vi "CAN Jaguar Get Status.vi"(8 "error in (no error)":errorcluster, 10 "Status Select":T1[](array[typedef])=[enum."Voltage"], 11 "CAN Jaguar Ref":T3={"Device Number"=0, "Control Mode"=enum."Percent VBus", "Inverted"=FALSE, "Semaphore"=refnum, "Max Vout"=12.0, "DevStatus"={"status"=FALSE, "code"=0, "source"=""}}) -> (0 "error out":errorcluster, 2 "Status":T2, 3 "CAN Jaguar Ref Out":T3={"Device Number"=0, "Control Mode"=enum."Percent VBus", "Inverted"=FALSE, "Semaphore"=refnum, "Max Vout"=12.0, "DevStatus"={"status"=FALSE, "code"=0, "source"=""}})   [LabVIEW 2009, in "CAN.lvlib"]
uses:
  CAN.lvlib
  SubVIs/CAN Jaguar Ref.ctl
  SubVIs/CAN Jaguar Control Mode.ctl
  SubVIs/CAN Jaguar Status.ctl
  SubVIs/CAN Jaguar Status Select.ctl
  SubVIs/CAN Motor Message IDs.ctl
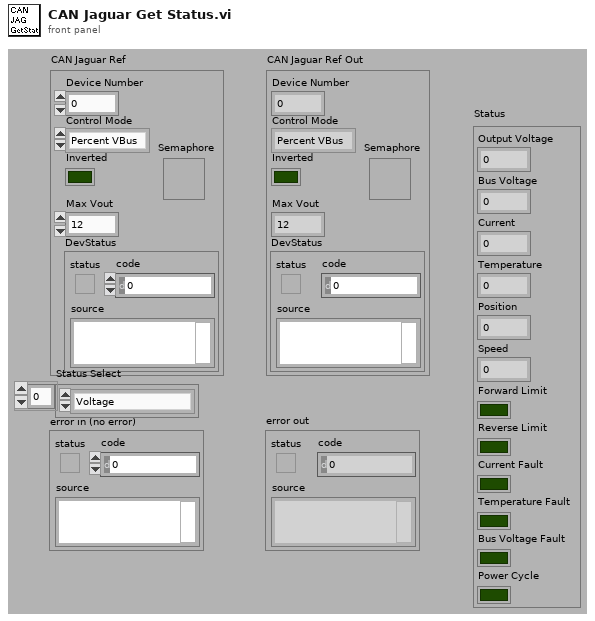
[diagram p1: front panel]
types:
  T1 = typedef "CAN.lvlib/CAN Jaguar Status Select.ctl" = enum16{"Voltage", "Current", "Temperature", "Position", "Speed", "Limit Switches", "Faults", "Power Cycle"}
  T2 = typedef "CAN.lvlib/CAN Jaguar Status.ctl" = cluster{"Output Voltage":dbl, "Bus Voltage":dbl, "Current":dbl, "Temperature":dbl, "Position":dbl, "Speed":dbl, "Forward Limit":bool, "Reverse Limit":bool, "Current Fault":bool, "Temperature Fault":bool, "Bus Voltage Fault":bool, "Power Cycle":bool}
  T3 = typedef "CAN.lvlib/CAN Jaguar Ref.ctl" = cluster{"Device Number":u8, "Control Mode":T4, "Inverted":bool, "Semaphore":T5, "Max Vout":dbl, "DevStatus":errorcluster}
  T4 = typedef "CAN.lvlib/CAN Jaguar Control Mode.ctl" = enum16{"Percent VBus", "Speed", "Position", "Current"}
  T5 = typedef "Semaphore RefNum" = refnum<k1>
  T6 = enum16{"big-endian, network order", "native, host order", "little-endian"}
  T7 = typedef "CAN Jaguar Status.ctl" = cluster{"Output Voltage":dbl, "Bus Voltage":dbl, "Current":dbl, "Temperature":dbl, "Position":dbl, "Speed":dbl, "Forward Limit":bool, "Reverse Limit":bool, "Current Fault":bool, "Temperature Fault":bool, "Bus Voltage Fault":bool, "Power Cycle":bool}
  T8 = typedef "CAN.lvlib/CAN Motor Message IDs.ctl" = u32
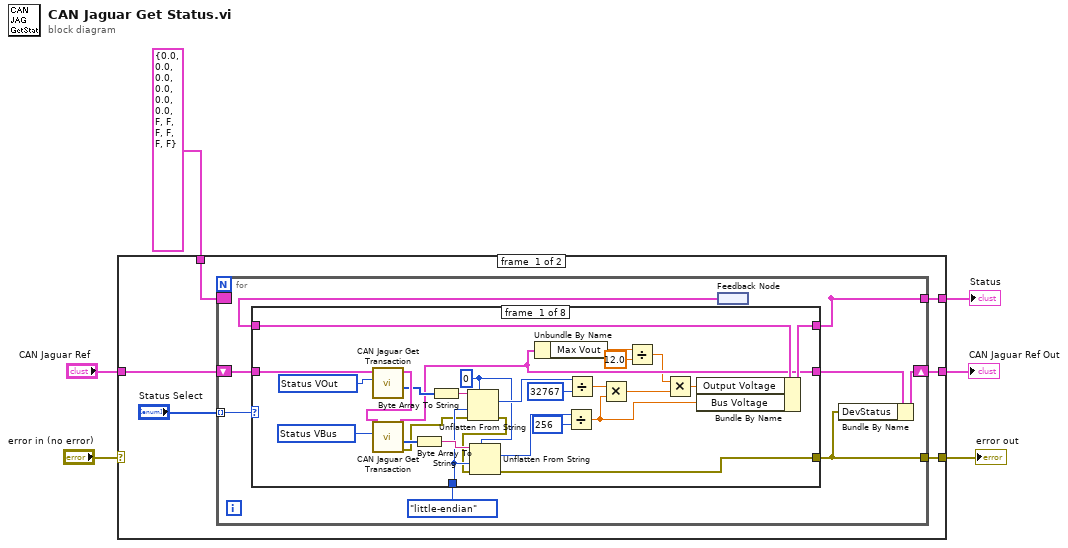
[diagram p0: block diagram]
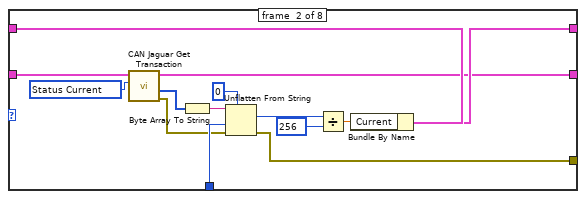
[diagram p2: hidden frame]
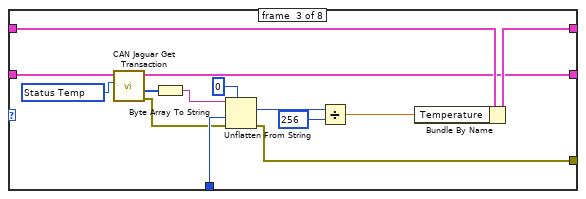
[diagram p3: hidden frame]
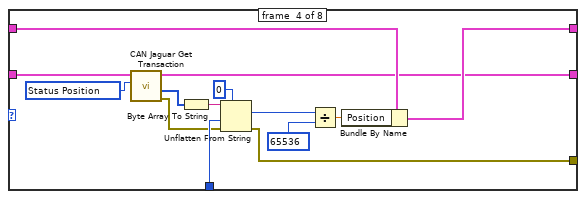
[diagram p4: hidden frame]
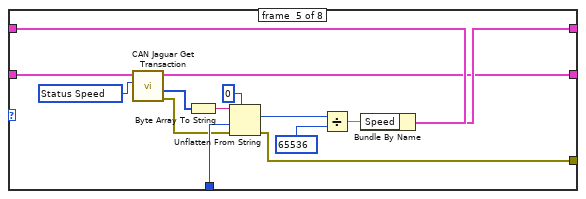
[diagram p5: hidden frame]
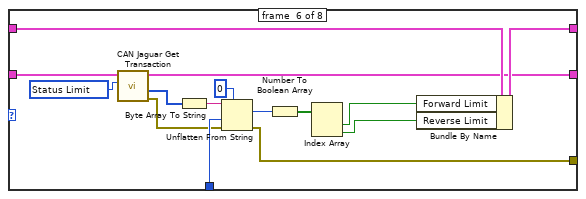
[diagram p6: hidden frame]
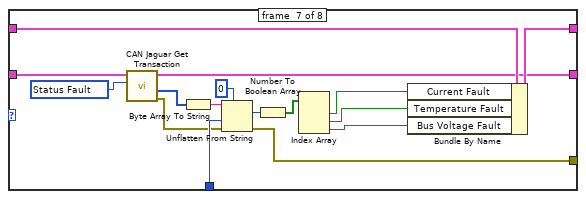
[diagram p7: hidden frame]
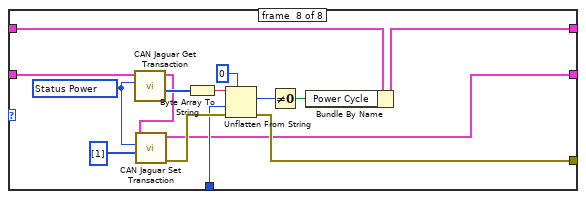
[diagram p8: hidden frame]
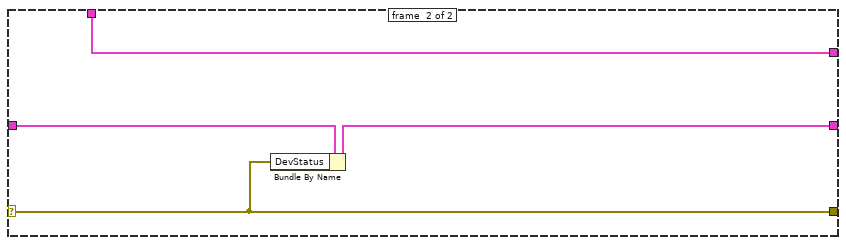
[diagram p9: hidden frame]
diagram:
  n1 = case shown="No Error" "error in (no error)" {
    selector: "error in (no error)" -> [_ w151]
    tunnel: [w7 w152] -> w6
    tunnel: "CAN Jaguar Ref" -> [w8 w153]
    tunnel: [w12 w151] -> w4
    tunnel: T2 {"Output Voltage"=0.0, "Bus Voltage"=0.0, "Current"=0.0, "Temperature"=0.0, "Position"=0.0, "Speed"=0.0, "Forward Limit"=FALSE, "Reverse Limit"=FALSE, "Current Fault"=FALSE, "Temperature Fault"=FALSE, "Bus Voltage Fault"=FALSE, "Power Cycle"=FALSE} ("Status") -> [w10 w150]
    tunnel: [w9 w150] -> w1
    frame #0 {
      n2 = for {
        tunnel: [w15] -> w12
        tunnel: "Status Select" -> [w20] mode=indexing
        border: w10 -> [_]
        tunnel: [w17] -> w9
        shift-right: [w13] -> w7
        shift-left: w8 -> [w16]
        n3 = feedback #1() -> (w19:T7)
        n4 = case shown="\"Voltage\"" w20 {
          tunnel: T6."little-endian" ("byte order (0:big-endian, network order)") -> [w29 w61 w75 w89 w103 w118 w134 w137]
          tunnel: [w47 w59 w73 w87 w101 w116 w132 w138] -> w15
          tunnel: w19 -> [w45 w58 w70 w86 w100 w115 w131 w149]
          tunnel: [w44 w57 w69 w85 w99 w114 w130 w148] -> w17
          tunnel: w16 -> [w34 w50 w67 w77 w91 w106 w121 w139]
          tunnel: [w25 w48 w62 w76 w90 w104 w119 w135] -> w14
          frame #0 {
            w27 = i16 0 ("Voltage")
            w35 = T8 33690624 items=["Volt Enable"=33685504, "Volt Disable"=33685568, "Volt Set"=33685632, "Volt Set Ramp"=33685696, "Speed Enable"=33686528, "Speed Disable"=33686592, "Speed Set"=33686656, "Speed P"=33686720, "Speed I"=33686784, "Speed D"=33686848, "Speed Ref"=33686912, "Position Enable"=33688576, "Position Disable"=33688640, "Position Set"=33688704, "Position P"=33688768, "Position I"=33688832, "Position D"=33688896, "Position Ref"=33688960, "Current Enable"=33689600, "Current Disable"=33689664, "Current Set"=33689728, "Current P"=33689792, "Current I"=33689856, "Current D"=33689920, "Status VOut"=33690624, "Status VBus"=33690688, "Status Current"=33690752, "Status Temp"=33690816, "Status Position"=33690880, "Status Speed"=33690944, "Status Limit"=33691008, "Status Fault"=33691072, "Status Power"=33691136, "Config Num Brushes"=33692672, "Config Encoder Lines"=33692736, "Config Pot Turns"=33692800, "Config Brake Coast"=33692864, "Config Limit Mode"=33692928, "Config Limit Fwd"=33692992, "Config Limit Rev"=33693056, "Config Max VOut"=33693120, "Config Fault Time"=33693184, "Motor Ack"=33693696] ("CAN Motor Message IDs")
            w36 = T8 33690688 items=["Volt Enable"=33685504, "Volt Disable"=33685568, "Volt Set"=33685632, "Volt Set Ramp"=33685696, "Speed Enable"=33686528, "Speed Disable"=33686592, "Speed Set"=33686656, "Speed P"=33686720, "Speed I"=33686784, "Speed D"=33686848, "Speed Ref"=33686912, "Position Enable"=33688576, "Position Disable"=33688640, "Position Set"=33688704, "Position P"=33688768, "Position I"=33688832, "Position D"=33688896, "Position Ref"=33688960, "Current Enable"=33689600, "Current Disable"=33689664, "Current Set"=33689728, "Current P"=33689792, "Current I"=33689856, "Current D"=33689920, "Status VOut"=33690624, "Status VBus"=33690688, "Status Current"=33690752, "Status Temp"=33690816, "Status Position"=33690880, "Status Speed"=33690944, "Status Limit"=33691008, "Status Fault"=33691072, "Status Power"=33691136, "Config Num Brushes"=33692672, "Config Encoder Lines"=33692736, "Config Pot Turns"=33692800, "Config Brake Coast"=33692864, "Config Limit Mode"=33692928, "Config Limit Fwd"=33692992, "Config Limit Rev"=33693056, "Config Max VOut"=33693120, "Config Fault Time"=33693184, "Motor Ack"=33693696] ("CAN Motor Message IDs")
            n5 = call "CAN Jaguar Get Transaction.vi"("Message ID"=w35, "CAN Jaguar Ref"=w34) -> ("Data"=w31:u8[], "CAN Jaguar Ref Out"=w33:T3)  [unwired: 1 in, 7 out]
            n6 = call "CAN Jaguar Get Transaction.vi"("Message ID"=w36, "CAN Jaguar Ref"=w33) -> ("error out"=w28:errorcluster, "Data"=w37:u8[], "CAN Jaguar Ref Out"=w25:T3)  [unwired: 1 in, 6 out]
            n7 = Byte Array To String(unsigned byte array=w37) -> (string=w38:string)
            n8 = Byte Array To String(unsigned byte array=w31) -> (string=w32:string)
            n9 = Unflatten From String(type=w27, binary string=w32, byte order (0:big-endian, network order)=w29, error in (no error)=w28) -> (value=w30:i16, error out=w26:errorcluster)  [unwired: 2 out]
            n10 = Unflatten From String(type=w27, binary string=w38, byte order (0:big-endian, network order)=w29, error in (no error)=w26) -> (value=w43:i16, error out=w47:errorcluster)  [unwired: 2 out]
            n11 = Unbundle By Name(w25) -> ("Max Vout"=w23:dbl)
            n12 = Divide(x=w43, y=i16 256) -> (x/y=w40:dbl)
            n13 = Divide(x=w30, y=i16 32767) -> (x/y=w39:dbl)
            n14 = Multiply(x=w39, y=w40) -> (x*y=w41:dbl)
            n15 = Divide(x=w23, y=12.0) -> (x/y=w21:dbl)
            n16 = Multiply(x=w21, y=w41) -> (x*y=w24:dbl)
            n17 = Bundle By Name(cluster=w45, "Output Voltage"=w24, "Bus Voltage"=w40) -> (w44:T7)
          }
          frame #1 {
            w49 = T8 33690752 items=["Volt Enable"=33685504, "Volt Disable"=33685568, "Volt Set"=33685632, "Volt Set Ramp"=33685696, "Speed Enable"=33686528, "Speed Disable"=33686592, "Speed Set"=33686656, "Speed P"=33686720, "Speed I"=33686784, "Speed D"=33686848, "Speed Ref"=33686912, "Position Enable"=33688576, "Position Disable"=33688640, "Position Set"=33688704, "Position P"=33688768, "Position I"=33688832, "Position D"=33688896, "Position Ref"=33688960, "Current Enable"=33689600, "Current Disable"=33689664, "Current Set"=33689728, "Current P"=33689792, "Current I"=33689856, "Current D"=33689920, "Status VOut"=33690624, "Status VBus"=33690688, "Status Current"=33690752, "Status Temp"=33690816, "Status Position"=33690880, "Status Speed"=33690944, "Status Limit"=33691008, "Status Fault"=33691072, "Status Power"=33691136, "Config Num Brushes"=33692672, "Config Encoder Lines"=33692736, "Config Pot Turns"=33692800, "Config Brake Coast"=33692864, "Config Limit Mode"=33692928, "Config Limit Fwd"=33692992, "Config Limit Rev"=33693056, "Config Max VOut"=33693120, "Config Fault Time"=33693184, "Motor Ack"=33693696] ("CAN Motor Message IDs")
            n18 = call "CAN Jaguar Get Transaction.vi"("Message ID"=w49, "CAN Jaguar Ref"=w50) -> ("error out"=w51:errorcluster, "Data"=w52:u8[], "CAN Jaguar Ref Out"=w48:T3)  [unwired: 1 in, 6 out]
            n19 = Byte Array To String(unsigned byte array=w52) -> (string=w53:string)
            n20 = Unflatten From String(type=i16 0 ("Voltage"), binary string=w53, byte order (0:big-endian, network order)=w61, error in (no error)=w51) -> (value=w56:i16, error out=w59:errorcluster)  [unwired: 2 out]
            n21 = Divide(x=w56, y=256) -> (x/y=w54:dbl)
            n22 = Bundle By Name(cluster=w58, "Current"=w54) -> (w57:T7)
          }
          frame #2 {
            w64 = T8 33690816 items=["Volt Enable"=33685504, "Volt Disable"=33685568, "Volt Set"=33685632, "Volt Set Ramp"=33685696, "Speed Enable"=33686528, "Speed Disable"=33686592, "Speed Set"=33686656, "Speed P"=33686720, "Speed I"=33686784, "Speed D"=33686848, "Speed Ref"=33686912, "Position Enable"=33688576, "Position Disable"=33688640, "Position Set"=33688704, "Position P"=33688768, "Position I"=33688832, "Position D"=33688896, "Position Ref"=33688960, "Current Enable"=33689600, "Current Disable"=33689664, "Current Set"=33689728, "Current P"=33689792, "Current I"=33689856, "Current D"=33689920, "Status VOut"=33690624, "Status VBus"=33690688, "Status Current"=33690752, "Status Temp"=33690816, "Status Position"=33690880, "Status Speed"=33690944, "Status Limit"=33691008, "Status Fault"=33691072, "Status Power"=33691136, "Config Num Brushes"=33692672, "Config Encoder Lines"=33692736, "Config Pot Turns"=33692800, "Config Brake Coast"=33692864, "Config Limit Mode"=33692928, "Config Limit Fwd"=33692992, "Config Limit Rev"=33693056, "Config Max VOut"=33693120, "Config Fault Time"=33693184, "Motor Ack"=33693696] ("CAN Motor Message IDs")
            n23 = call "CAN Jaguar Get Transaction.vi"("Message ID"=w64, "CAN Jaguar Ref"=w67) -> ("error out"=w63:errorcluster, "Data"=w66:u8[], "CAN Jaguar Ref Out"=w62:T3)  [unwired: 1 in, 6 out]
            n24 = Byte Array To String(unsigned byte array=w66) -> (string=w65:string)
            n25 = Unflatten From String(type=i16 0 ("Voltage"), binary string=w65, byte order (0:big-endian, network order)=w75, error in (no error)=w63) -> (value=w72:i16, error out=w73:errorcluster)  [unwired: 2 out]
            n26 = Divide(x=w72, y=256) -> (x/y=w68:dbl)
            n27 = Bundle By Name(cluster=w70, "Temperature"=w68) -> (w69:T7)
          }
          frame #3 {
            w80 = T8 33690880 items=["Volt Enable"=33685504, "Volt Disable"=33685568, "Volt Set"=33685632, "Volt Set Ramp"=33685696, "Speed Enable"=33686528, "Speed Disable"=33686592, "Speed Set"=33686656, "Speed P"=33686720, "Speed I"=33686784, "Speed D"=33686848, "Speed Ref"=33686912, "Position Enable"=33688576, "Position Disable"=33688640, "Position Set"=33688704, "Position P"=33688768, "Position I"=33688832, "Position D"=33688896, "Position Ref"=33688960, "Current Enable"=33689600, "Current Disable"=33689664, "Current Set"=33689728, "Current P"=33689792, "Current I"=33689856, "Current D"=33689920, "Status VOut"=33690624, "Status VBus"=33690688, "Status Current"=33690752, "Status Temp"=33690816, "Status Position"=33690880, "Status Speed"=33690944, "Status Limit"=33691008, "Status Fault"=33691072, "Status Power"=33691136, "Config Num Brushes"=33692672, "Config Encoder Lines"=33692736, "Config Pot Turns"=33692800, "Config Brake Coast"=33692864, "Config Limit Mode"=33692928, "Config Limit Fwd"=33692992, "Config Limit Rev"=33693056, "Config Max VOut"=33693120, "Config Fault Time"=33693184, "Motor Ack"=33693696] ("CAN Motor Message IDs")
            n28 = call "CAN Jaguar Get Transaction.vi"("Message ID"=w80, "CAN Jaguar Ref"=w77) -> ("error out"=w79:errorcluster, "Data"=w78:u8[], "CAN Jaguar Ref Out"=w76:T3)  [unwired: 1 in, 6 out]
            n29 = Byte Array To String(unsigned byte array=w78) -> (string=w81:string)
            n30 = Unflatten From String(type=0 ("Voltage"), binary string=w81, byte order (0:big-endian, network order)=w89, error in (no error)=w79) -> (value=w84:i32, error out=w87:errorcluster)  [unwired: 2 out]
            n31 = Divide(x=w84, y=65536 ("value")) -> (x/y=w83:dbl)
            n32 = Bundle By Name(cluster=w86, "Position"=w83) -> (w85:T7)
          }
          frame #4 {
            w92 = T8 33690944 items=["Volt Enable"=33685504, "Volt Disable"=33685568, "Volt Set"=33685632, "Volt Set Ramp"=33685696, "Speed Enable"=33686528, "Speed Disable"=33686592, "Speed Set"=33686656, "Speed P"=33686720, "Speed I"=33686784, "Speed D"=33686848, "Speed Ref"=33686912, "Position Enable"=33688576, "Position Disable"=33688640, "Position Set"=33688704, "Position P"=33688768, "Position I"=33688832, "Position D"=33688896, "Position Ref"=33688960, "Current Enable"=33689600, "Current Disable"=33689664, "Current Set"=33689728, "Current P"=33689792, "Current I"=33689856, "Current D"=33689920, "Status VOut"=33690624, "Status VBus"=33690688, "Status Current"=33690752, "Status Temp"=33690816, "Status Position"=33690880, "Status Speed"=33690944, "Status Limit"=33691008, "Status Fault"=33691072, "Status Power"=33691136, "Config Num Brushes"=33692672, "Config Encoder Lines"=33692736, "Config Pot Turns"=33692800, "Config Brake Coast"=33692864, "Config Limit Mode"=33692928, "Config Limit Fwd"=33692992, "Config Limit Rev"=33693056, "Config Max VOut"=33693120, "Config Fault Time"=33693184, "Motor Ack"=33693696] ("CAN Motor Message IDs")
            n33 = call "CAN Jaguar Get Transaction.vi"("Message ID"=w92, "CAN Jaguar Ref"=w91) -> ("error out"=w93:errorcluster, "Data"=w94:u8[], "CAN Jaguar Ref Out"=w90:T3)  [unwired: 1 in, 6 out]
            n34 = Byte Array To String(unsigned byte array=w94) -> (string=w95:string)
            n35 = Unflatten From String(type=0 ("Voltage"), binary string=w95, byte order (0:big-endian, network order)=w103, error in (no error)=w93) -> (value=w96:i32, error out=w101:errorcluster)  [unwired: 2 out]
            n36 = Divide(x=w96, y=65536 ("value")) -> (x/y=w97:dbl)
            n37 = Bundle By Name(cluster=w100, "Speed"=w97) -> (w99:T7)
          }
          frame #5 {
            w105 = T8 33691008 items=["Volt Enable"=33685504, "Volt Disable"=33685568, "Volt Set"=33685632, "Volt Set Ramp"=33685696, "Speed Enable"=33686528, "Speed Disable"=33686592, "Speed Set"=33686656, "Speed P"=33686720, "Speed I"=33686784, "Speed D"=33686848, "Speed Ref"=33686912, "Position Enable"=33688576, "Position Disable"=33688640, "Position Set"=33688704, "Position P"=33688768, "Position I"=33688832, "Position D"=33688896, "Position Ref"=33688960, "Current Enable"=33689600, "Current Disable"=33689664, "Current Set"=33689728, "Current P"=33689792, "Current I"=33689856, "Current D"=33689920, "Status VOut"=33690624, "Status VBus"=33690688, "Status Current"=33690752, "Status Temp"=33690816, "Status Position"=33690880, "Status Speed"=33690944, "Status Limit"=33691008, "Status Fault"=33691072, "Status Power"=33691136, "Config Num Brushes"=33692672, "Config Encoder Lines"=33692736, "Config Pot Turns"=33692800, "Config Brake Coast"=33692864, "Config Limit Mode"=33692928, "Config Limit Fwd"=33692992, "Config Limit Rev"=33693056, "Config Max VOut"=33693120, "Config Fault Time"=33693184, "Motor Ack"=33693696] ("CAN Motor Message IDs")
            n38 = call "CAN Jaguar Get Transaction.vi"("Message ID"=w105, "CAN Jaguar Ref"=w106) -> ("error out"=w108:errorcluster, "Data"=w107:u8[], "CAN Jaguar Ref Out"=w104:T3)  [unwired: 1 in, 6 out]
            n39 = Byte Array To String(unsigned byte array=w107) -> (string=w109:string)
            n40 = Unflatten From String(type=u8 0 ("Voltage"), binary string=w109, byte order (0:big-endian, network order)=w118, error in (no error)=w108) -> (value=w113:u8, error out=w116:errorcluster)  [unwired: 2 out]
            n41 = Number To Boolean Array(number=w113) -> (Boolean array=w112:bool[])
            n42 = Index Array(array=w112) -> (element #1=w111:bool, element #2=w110:bool)  [unwired: 2 in]
            n43 = Bundle By Name(cluster=w115, "Forward Limit"=w111, "Reverse Limit"=w110) -> (w114:T7)
          }
          frame #6 {
            w120 = T8 33691072 items=["Volt Enable"=33685504, "Volt Disable"=33685568, "Volt Set"=33685632, "Volt Set Ramp"=33685696, "Speed Enable"=33686528, "Speed Disable"=33686592, "Speed Set"=33686656, "Speed P"=33686720, "Speed I"=33686784, "Speed D"=33686848, "Speed Ref"=33686912, "Position Enable"=33688576, "Position Disable"=33688640, "Position Set"=33688704, "Position P"=33688768, "Position I"=33688832, "Position D"=33688896, "Position Ref"=33688960, "Current Enable"=33689600, "Current Disable"=33689664, "Current Set"=33689728, "Current P"=33689792, "Current I"=33689856, "Current D"=33689920, "Status VOut"=33690624, "Status VBus"=33690688, "Status Current"=33690752, "Status Temp"=33690816, "Status Position"=33690880, "Status Speed"=33690944, "Status Limit"=33691008, "Status Fault"=33691072, "Status Power"=33691136, "Config Num Brushes"=33692672, "Config Encoder Lines"=33692736, "Config Pot Turns"=33692800, "Config Brake Coast"=33692864, "Config Limit Mode"=33692928, "Config Limit Fwd"=33692992, "Config Limit Rev"=33693056, "Config Max VOut"=33693120, "Config Fault Time"=33693184, "Motor Ack"=33693696] ("CAN Motor Message IDs")
            n44 = call "CAN Jaguar Get Transaction.vi"("Message ID"=w120, "CAN Jaguar Ref"=w121) -> ("error out"=w123:errorcluster, "Data"=w122:u8[], "CAN Jaguar Ref Out"=w119:T3)  [unwired: 1 in, 6 out]
            n45 = Byte Array To String(unsigned byte array=w122) -> (string=w124:string)
            n46 = Unflatten From String(type=u16 0 ("Voltage"), binary string=w124, byte order (0:big-endian, network order)=w134, error in (no error)=w123) -> (value=w129:u16, error out=w132:errorcluster)  [unwired: 2 out]
            n47 = Number To Boolean Array(number=w129) -> (Boolean array=w128:bool[])
            n48 = Index Array(array=w128) -> (element #1=w127:bool, element #2=w126:bool, element #3=w125:bool)  [unwired: 3 in]
            n49 = Bundle By Name(cluster=w131, "Current Fault"=w127, "Temperature Fault"=w126, "Bus Voltage Fault"=w125) -> (w130:T7)
          }
          frame #7 {
            w144 = T8 33691136 items=["Volt Enable"=33685504, "Volt Disable"=33685568, "Volt Set"=33685632, "Volt Set Ramp"=33685696, "Speed Enable"=33686528, "Speed Disable"=33686592, "Speed Set"=33686656, "Speed P"=33686720, "Speed I"=33686784, "Speed D"=33686848, "Speed Ref"=33686912, "Position Enable"=33688576, "Position Disable"=33688640, "Position Set"=33688704, "Position P"=33688768, "Position I"=33688832, "Position D"=33688896, "Position Ref"=33688960, "Current Enable"=33689600, "Current Disable"=33689664, "Current Set"=33689728, "Current P"=33689792, "Current I"=33689856, "Current D"=33689920, "Status VOut"=33690624, "Status VBus"=33690688, "Status Current"=33690752, "Status Temp"=33690816, "Status Position"=33690880, "Status Speed"=33690944, "Status Limit"=33691008, "Status Fault"=33691072, "Status Power"=33691136, "Config Num Brushes"=33692672, "Config Encoder Lines"=33692736, "Config Pot Turns"=33692800, "Config Brake Coast"=33692864, "Config Limit Mode"=33692928, "Config Limit Fwd"=33692992, "Config Limit Rev"=33693056, "Config Max VOut"=33693120, "Config Fault Time"=33693184, "Motor Ack"=33693696] ("CAN Motor Message IDs")
            n50 = call "CAN Jaguar Get Transaction.vi"("Message ID"=w144, "CAN Jaguar Ref"=w139) -> ("Data"=w145:u8[], "CAN Jaguar Ref Out"=w136:T3)  [unwired: 1 in, 7 out]
            n51 = call "CAN Jaguar Set Transaction.vi"("Data"=u8[] [1] ("data"), "Message ID"=w144, "CAN Jaguar Ref"=w136) -> ("error out"=w146:errorcluster, "CAN Jaguar Ref Out"=w135:T3)  [unwired: 1 in, 6 out]
            n52 = Byte Array To String(unsigned byte array=w145) -> (string=w141:string)
            n53 = Unflatten From String(type=u8 0 ("Voltage"), binary string=w141, byte order (0:big-endian, network order)=w137, error in (no error)=w146) -> (value=w140:u8, error out=w138:errorcluster)  [unwired: 2 out]
            n54 = Not Equal To 0?(x=w140) -> (x != 0?=w147:bool)
            n55 = Bundle By Name(cluster=w149, "Power Cycle"=w147) -> (w148:T7)
          }
        }
        n56 = Bundle By Name(cluster=w14, "DevStatus"=w15) -> (w13:T3)
      }
    }
    frame #1 {
      n57 = Bundle By Name(cluster=w153, "DevStatus"=w151) -> (w152:T3)
    }
  }
  "CAN Jaguar Ref Out" <- w6
  "error out" <- w4
  "Status" <- w1
